vi "Clip Image.vi"(8 "error in (no error)":errorcluster, 10 "ROI":T1 {"Rotation" format="%.2f"; "Left" scale=0.0..1024.0; "Right" scale=0.0..1024.0}, 11 "Actor in":refnum<class "Actor.lvclass">) -> (0 "error out":errorcluster, 3 "Actor out":refnum<class "Actor.lvclass">)   [LabVIEW 2015, in "Actor.lvclass"]
uses:
  Actor.lvclass
  Actor.lvclass/Actor.ctl
  ImageOperaion/ImageOperation.lvclass
  FileOperation/FileOperation.lvclass
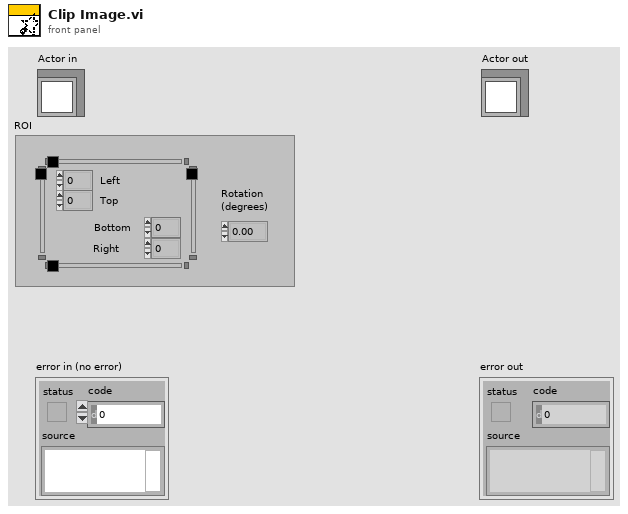
[diagram p1: front panel]
types:
  T1 = typedef "IMAQ Rectangle" = cluster{"Left":i32, "Top":i32, "Right":i32, "Bottom":i32, "Rotation":dbl}
  T2 = typedef "IMAQ Image.ctl" = refnum<image>
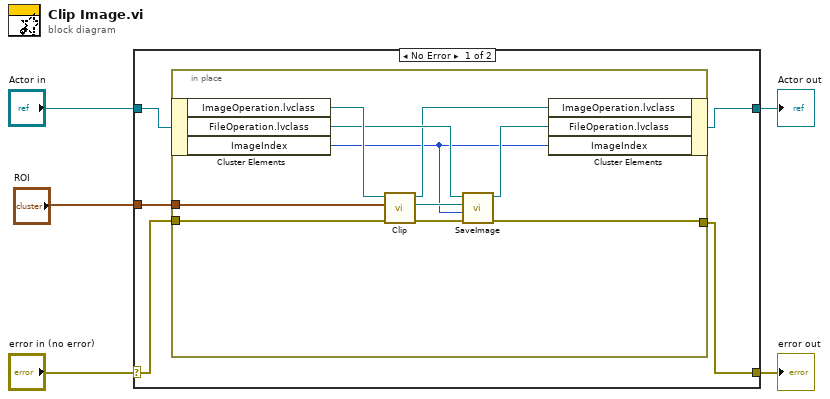
[diagram p0: block diagram]
diagram:
  n1 = case shown="No Error" "error in (no error)" {
    selector: "error in (no error)" -> [w8 w22]
    tunnel: [w6 w22] -> w4
    tunnel: [w7 w21] -> w2
    tunnel: "Actor in" -> [w9 w21]
    tunnel: "ROI" -> [w10 _]
    frame No Error {
      n2 = in-place {
        in-place-border: w10 -> [w20]
        in-place-border: w8 -> [w18]
        in-place-border: [w11] -> w6
        n3 = in-place-cluster #1(w9) -> ("ImageOperation.lvclass"=w19:refnum<class "ImageOperation.lvclass">, "FileOperation.lvclass"=w17:refnum<class "FileOperation.lvclass">, "ImageIndex"=w12:i32)
        n4 = call "Clip.vi"("error in (no error)"=w18, "ROI"=w20, "ImageOperation in"=w19) -> ("error out"=w14:errorcluster, "Image Dst Out"=w16:T2, "ImageOperation out"=w15:refnum<class "ImageOperation.lvclass">)  [unwired: 6 in]
        n5 = call "SaveImage.vi"("error in (no error)"=w14, "IndexOfImages"=w12, "Image Dst In"=w16, "FileOperation in"=w17) -> ("error out"=w11:errorcluster, "FileOperation out"=w13:refnum<class "FileOperation.lvclass">)  [unwired: 6 in]
        n6 = in-place-cluster #1("ImageOperation.lvclass"=w15, "FileOperation.lvclass"=w13, "ImageIndex"=w12) -> (w7:refnum<class "Actor.lvclass">)
      }
    }
    frame Error {
    }
  }
  "error out" <- w4
  "Actor out" <- w2
